vi "KoherasInterfaceGetFGV.vi"(8 "in":errorcluster, 10 "Set_Get":enum16{"Set", "Get"}(ring), 11 "in":refnum<visa-resource-name>="COM3") -> (0 "out":errorcluster, 3 "out":refnum<visa-resource-name>)   [LabVIEW 2011]
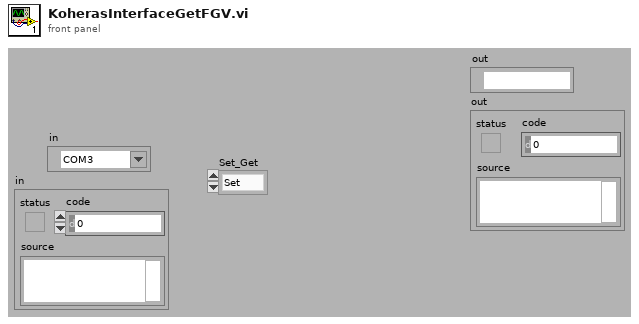
[diagram p1: front panel]
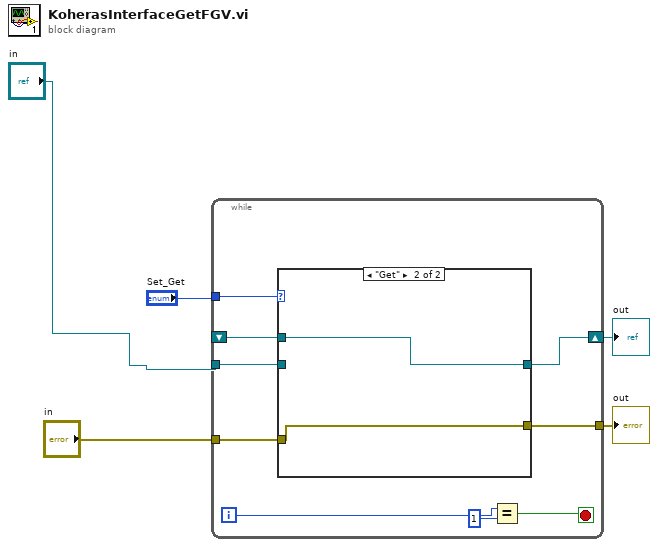
[diagram p0: block diagram]
diagram:
  n1 = while {
    tunnel: "Set_Get" -> [w14]
    tunnel: "in" -> [w13]
    shift-right: [w12] -> w3
    shift-left: _ -> [w11]
    tunnel: [w7] -> w1
    tunnel: "in" -> [w6]
    i -> [w9]
    stop <- w10 stop-if-true
    n2 = case shown="\"Get\"" w14 {
      tunnel: w13 -> [w15 _]
      tunnel: [w15 w17] -> w12
      tunnel: w11 -> [_ w17]
      tunnel: [_ w16] -> w7
      tunnel: w6 -> [_ w16]
      frame "Set", Default {
      }
      frame "Get" {
      }
    }
    n3 = Equal?(x=w9, y=1) -> (x = y?=w10:bool)
  }
  "out" <- w3
  "out" <- w1
